vi "GetFrequencyValue.vi"(0 "PM Cmds In":refnum<k24>, 5 "Device Key In":string, 11 "error in":errorcluster) -> (4 "PM Cmds Out":refnum<k24>, 6 "Device Key Out":string, 8 "I/O Status":i32, 10 "Frequency Value":dbl format="%^#_6g", 15 "error out":errorcluster)   [LabVIEW 2010]
uses:
  C:/Code/Apps/Utilities/PM2935/PMWinApp/PM_Installer/Master/Samples/1918 - 2936 Family/LabVIEW/LabVIEW 2010/PowerMeterCommands.dll
  PowerMeterCommands.dll
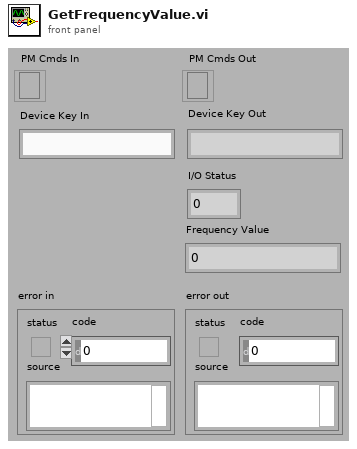
[diagram p1: front panel]
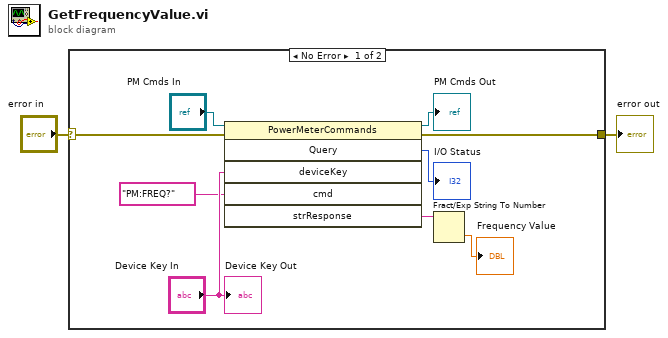
[diagram p0: block diagram]
diagram:
  n1 = case shown="No Error" "error in" {
    selector: "error in" -> [w8 w12]
    tunnel: [w10 w12] -> w2
    frame No Error {
      n2 = invoke class="PowerMeterCommands" method="Query"(reference="PM Cmds In", error in=w8, "deviceKey"="Device Key In", "cmd"="PM:FREQ?") -> (reference out=→"PM Cmds Out":refnum<k24>, error out=w10:errorcluster, "Query"=→"I/O Status":i32, "strResponse"=w4:string)  [unwired: 2 in, 2 out]
      n3 = Fract/Exp String To Number(string=w4) -> (number=→"Frequency Value":dbl)  [unwired: 3 in, 1 out]
      "Device Key Out" <- "Device Key In"
    }
    frame Error {
    }
  }
  "error out" <- w2
